vi "pressure calibration.vi"(11 "input variable":dbl) -> (3 "output variable":dbl)   [LabVIEW 2020]
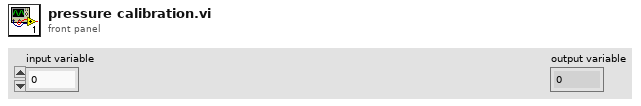
[diagram p1: front panel]
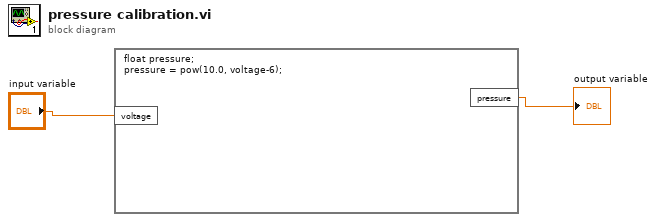
[diagram p0: block diagram]
diagram:
  n1 = formula code="float pressure;\npressure = pow(10.0, voltage-6);"("voltage"="input variable") -> ("pressure"=→"output variable":dbl)
